vi "CalibrateDistanceCameraSyringe (SubVI).vi"() -> ()   [LabVIEW 2016]
uses:
  <vilib>/LabVIEW Interface for Arduino/Type Defs/Arduino Resource.ctl
  <vilib>/LabVIEW Interface for Arduino/Type Defs/Board Type.ctl
  C:/Users/Aerotech/Documents/BNL_ThermomechanicalStave/AerotechLibraries/Bin/Aerotech.A3200.dll
  AerotechLibraries/Bin/Aerotech.A3200.dll
  <vilib>/vision/Measure.llb/Edge Options.ctl
  <vilib>/vision/Measure.llb/Edge Polarity.ctl
  <vilib>/vision/Image Controls.llb/IMAQ Image.ctl
  <vilib>/LabVIEW Interface for Arduino/Type Defs/Pin Mode.ctl
  <vilib>/LabVIEW Interface for Arduino/LabVIEW Interface for Arduino.lvlib
  <vilib>/vision/NI_Vision_Development_Module.lvlib
panel:
  in  "?":T1(tab)
  in  "Coordinate to Dot":T2={"X [mm]"=10.0, "Y [mm]"=-20.0, "Z [mm] "=43.0}
  in  "Estimate distance x":dbl
  in  "Estimate distance y":dbl
  in  "Camera Z":dbl
  out "XYZ Stage Control":refnum<k24>
  out "Arduino Resource":T3={"VISA resource"="COM3", "Board Type"=enum."Uno", "Connection Type"=enum."USB / Serial", "Bytes Per Packet (15)"=15}
  in  "Digital I/O Pin":u8=7
  in  "Axis speeds (mm/s)":T5={"vX [mm]"=150.0, "vY [mm]"=150.0, "vZ [mm] "=150.0}
  in  "Lowest Z Position":dbl=46.0
  in  "um/pix resolution":dbl=1.5800403213058958
  out "Template Image":T6
  in  "Template Path":path=path "C:/Users/Aerotech/Documents/BNL_ThermomechanicalStave/0_Calibration"
  in  "Circle Finding Options":T9={"Search  Direction"=1, "Edge Options"={"Edge Polarity"=2, "Kernel Size"=3, "Width"=3, "Minimum Edge Strength"=10.0, "Interpolation Type"=enum."Bilinear Fixed", "Data Processing Method"=enum."Median"}, "Show Search Area"=FALSE, "Show Search Lines"=FALSE, "Show Edges Found"=FALSE, "Show Result"=TRUE, "Search Area Color"=65280, "Search Lines Color"=255, "Edge Locations Color"=16776960, "Result Color"=65511, "Overlay Group Name"=""} {"Search  Direction" items=["Outside to Inside", "Inside to Outside"]; "Edge Options"."Edge Polarity" items=["All Edges", "Rising Edges", "Falling Edges"]; "Edge Options"."Minimum Edge Strength" format="%.2f"; "Edge Options"."Width" step=2; "Edge Options"."Kernel Size" step=2}
  in  "Circle ROI Descriptor":T10={"Global Rectangle"=[675, 567, 1751, 1642], "Contours"=[{"ID"=enum."External", "Type"=7, "Coordinates"=[1212, 1104, 85, 537, 0, 0]}]} {"Contours"."Type" items=["No Selection", "Point", "Line", "Rectangle", "Oval", "Polygon", "Freehand Region", "Annulus", "Unused2", "Unused3", "Broken Line", "Freehand Line", "Rotated Rectangle"]}
  in  "Pattern Match Settings":T11={"Algorithm"=2, "Number of Matches Requested"=1, "Minimum Match Score"=700.0, "SubPixel Accuracy"=TRUE, "Rotation Angle Ranges"=[{"Start"=0.0, "End"=360.0}], "Show Search Area"=FALSE, "Show Result"=TRUE} {"Rotation Angle Ranges"."End" format="%.1f"; "Rotation Angle Ranges"."Start" format="%.1f"; "Minimum Match Score" min=0 max=1000 format="%.2f"; "Number of Matches Requested" min=1; "Algorithm" items=["All", "Low Discrepancy Sampling", "Grayscale Value Pyramid", "Gradients Pyramid"]}
  in  "Circle Fit Options":T12={"Process"=enum."Get Best Edge", "Step Size"=3.0, "Max Pixel Radius"=3}
  out "Estimate location":T2={"X [mm]"=10.0, "Y [mm]"=-20.0, "Z [mm] "=43.0}
  out "X/Y difference (CAMERA - SYRINGE)":dbl[](array[numeric])
  out "error out":errorcluster
  out "pixels x":dbl=1920.0
  out "pixels y":dbl=1374.0
  out "Dot image":T6(plugin-control)
  in  "error in":errorcluster
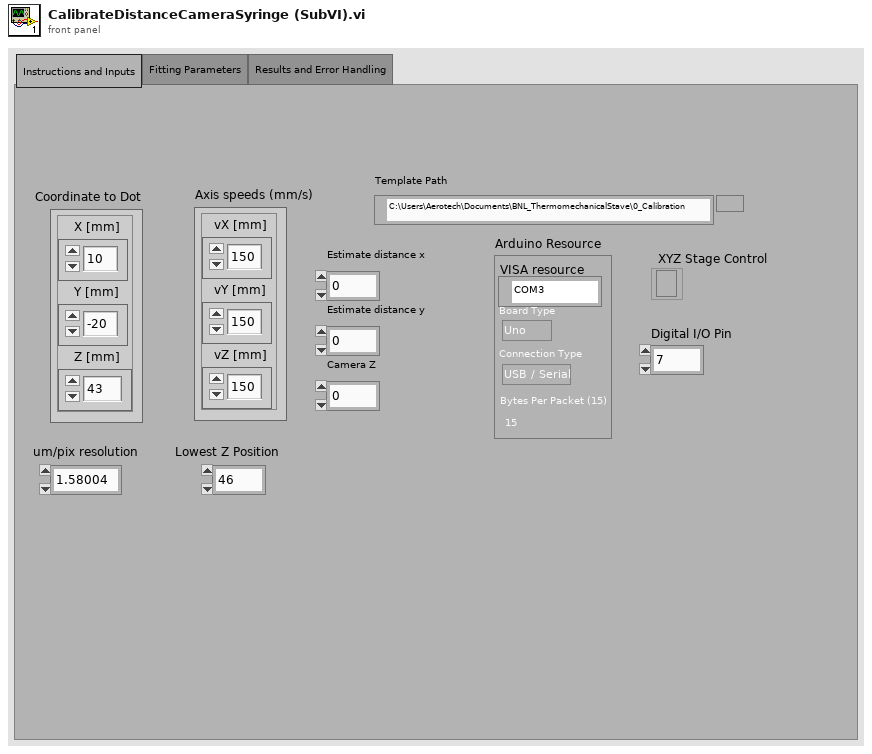
[diagram p1: front panel]
types:
  T1 = enum32{"Instructions and Inputs", "Fitting Parameters", "Results and Error Handling"}
  T2 = cluster{"X [mm]":dbl, "Y [mm]":dbl, "Z [mm] ":dbl}
  T3 = typedef "LabVIEW Interface for Arduino.lvlib/Arduino Resource.ctl" = cluster{"VISA resource":refnum<visa-resource-name>, "Board Type":T4, "Connection Type":enum8{"USB / Serial"}, "Bytes Per Packet (15)":u8}
  T4 = typedef "LabVIEW Interface for Arduino.lvlib/Board Type.ctl" = enum16{"Uno", "Dimuelanove w/Atmega 328", "Mega 2560"}
  T5 = cluster{"vX [mm]":dbl, "vY [mm]":dbl, "vZ [mm] ":dbl}
  T6 = typedef "IMAQ Image.ctl" = refnum<image>
  T7 = typedef "Edge Options.ctl" = cluster{"Edge Polarity":T8, "Kernel Size":u32, "Width":u32, "Minimum Edge Strength":sgl, "Interpolation Type":enum32{"Zero Order", "Bilinear", "Quadratic", "Cubic", "Bilinear Fixed"}, "Data Processing Method":enum32{"Average", "Median"}}
  T8 = typedef "Edge Polarity.ctl" = u32
  T9 = cluster{"Search  Direction":u32, "Edge Options":T7, "Show Search Area":bool, "Show Search Lines":bool, "Show Edges Found":bool, "Show Result":bool, "Search Area Color":u32, "Search Lines Color":u32, "Edge Locations Color":u32, "Result Color":u32, "Overlay Group Name":string}
  T10 = cluster{"Global Rectangle":i32[], "Contours":cluster{"ID":enum32{"External", "Internal"}, "Type":u32, "Coordinates":i32[]}[]}
  T11 = cluster{"Algorithm":i32, "Number of Matches Requested":i32, "Minimum Match Score":sgl, "SubPixel Accuracy":bool, "Rotation Angle Ranges":cluster{"Start":sgl, "End":sgl}[], "Show Search Area":bool, "Show Result":bool}
  T12 = cluster{"Process":enum16{"Get First Edge", "Get First + Last Edge", "Get All Edges", "Get Best Edge"}, "Step Size":dbl, "Max Pixel Radius":i32}
  T13 = typedef "Image Type" = u32
  T14 = typedef "LabVIEW Interface for Arduino.lvlib/Pin Mode.ctl" = enum8{"Input", "Output"}
  T15 = cluster{"Final X":dbl, "Final Y":dbl, "Final Z":dbl}
  T16 = cluster{"X [mm]":dbl, "Y [mm]":dbl, "Lowest Z Position":dbl}
  T17 = cluster{"Position":cluster{"x":sgl, "y":sgl}, "Angle":sgl, "Scale":sgl, "Score":sgl, "Bounding Box":cluster{"x":sgl, "y":sgl}[]}[]
  T18 = cluster{"Global Rectangle":i32[], cluster{"ID":enum32{"External", "Internal"}, "Type":u32, "Coordinates":i32[]}[]}
  T19 = cluster{"Center (Pixels)":cluster{"X":sgl, "Y":sgl}, "Radius (Pixels)":dbl, "Center (Real-World)":cluster{"X":sgl, "Y":sgl}, "Radius (Real-World)":dbl, "Roundness (Real-World)":dbl, "Average Strength":dbl, "Average SNR (dB)":dbl}
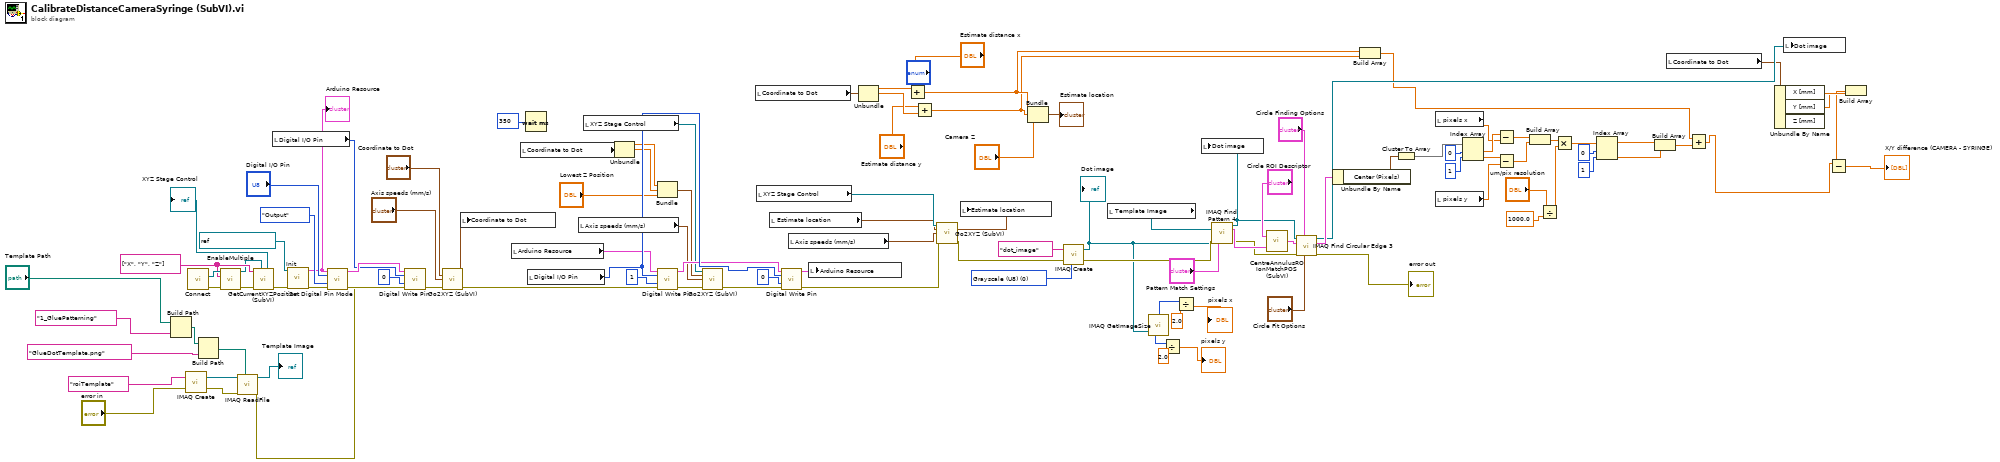
[diagram p0: block diagram]
diagram:
  w64 = T13 0 items=["Grayscale (U8)", "Grayscale (I16)", "Grayscale (SGL)", "Complex (CSG)", "RGB (U32)", "HSL (U32)", "RGB (U64)", "Grayscale (U16)"] ("Image Type")
  w100 = string[] ["X", "Y", "Z"] ("Axes Names")
  n1 = Build Path(base path="Template Path", name or relative path="1_GluePatterning") -> (appended path=w9:path)
  n2 = call "IMAQ Create"("Image Name"="roiTemplate", "error in (no error)"="error in") -> ("New Image"=w12:T6, "error out"=w13:errorcluster)  [unwired: 3 in]
  n3 = Build Path(base path=w9, name or relative path="GlueDotTemplate.png") -> (appended path=w7:path)
  n4 = call "IMAQ ReadFile"("File Path"=w7, "error in (no error)"=w13, "Image"=w12) -> ("error out"=w4:errorcluster, "Image Out"=→"Template Image":T6)  [unwired: 4 in, 3 out]
  n5 = call "Connect.vi"("error in (no error)"=w4) -> ("error out"=w102:errorcluster, "controller"=w101:refnum<k24>)  [unwired: 9 in]
  n6 = call "EnableMultiple.vi"("error in (no error)"=w102, "axis names"=w100, "controller in"=w101) -> ("error out"=w103:errorcluster, "controller out"=w99:refnum<k24>)  [unwired: 7 in]
  n7 = call "GetCurrentXYZPosition (SubVI).vi"(".NET Refnum in - Device"=w99, "error in (no error)"=w103, "Axes Names"=w100) -> ("error out"=w97:errorcluster, ".NET Refnum out  - Device"=→"XYZ Stage Control":refnum<k24>)  [unwired: 3 in, 4 out]
  n8 = local read "Digital I/O Pin"() -> (w105:u8)
  n9 = call <vilib>:"Init.vi"("VISA resource"=refnum<visa-resource-name> "COM3", "error in"=w97) -> ("Arduino Resource"=w104:T3, "error out"=w106:errorcluster)  [unwired: 16 in]
  "Arduino Resource" <- w104
  n10 = call <vilib>:"Set Digital Pin Mode.vi"("Arduino Resource"=w104, "Digital I/O Pin"="Digital I/O Pin", "Pin Mode (Input)"=Pin_Mode."Output", "error in"=w106) -> ("Arduino Resource"=w109:T3, "error out"=w110:errorcluster)  [unwired: 10 in]
  n11 = call <vilib>:"Digital Write Pin.vi"("Arduino Resource"=w109, "Digital I/O Pin (0)"=w105, "Value (0)"=u8 0, "error in"=w110) -> ("error out"=w94:errorcluster)  [unwired: 10 in, 1 out]
  n12 = call "Go2XYZ (SubVI).vi"("Go to Coordinates"="Coordinate to Dot", "Axis Speeds"="Axis speeds (mm/s)", "error in (no error)"=w94) -> ("Final Position"=w61:T15, "error out"=w90:errorcluster)  [unwired: 8 in, 3 out]
  n13 = local write "Coordinate to Dot"(w61) -> ()
  n14 = local read "Arduino Resource"() -> (w82:T3)
  n15 = local read "Coordinate to Dot"() -> (w85:T2)
  n16 = Wait (ms)(milliseconds to wait=u32 350) -> ()  [unwired: 1 out]
  n17 = local read "Digital I/O Pin"() -> (w92:u8)
  n18 = local read "Axis speeds (mm/s)"() -> (w88:T5)
  n19 = local read "XYZ Stage Control"() -> (w87:refnum<k24>)
  n20 = Unbundle(w85) -> ("X [mm]"=w84:dbl, "Y [mm]"=w83:dbl)  [unwired: 1 out]
  n21 = Bundle("X [mm]"=w84, "Y [mm]"=w83, "Lowest Z Position"="Lowest Z Position") -> (w86:T16)  [unwired: 1 in]
  n22 = call <vilib>:"Digital Write Pin.vi"("Arduino Resource"=w82, "Digital I/O Pin (0)"=w92, "Value (0)"=u8 1, "error in"=w90) -> ("Arduino Resource"=w91:T3, "error out"=w80:errorcluster)  [unwired: 10 in]
  n23 = call "Go2XYZ (SubVI).vi"(".NET Refnum in"=w87, "Go to Coordinates"=w86, "Axis Speeds"=w88, "error in (no error)"=w80) -> ("error out"=w93:errorcluster)  [unwired: 7 in, 4 out]
  n24 = local read "Coordinate to Dot"() -> (w78:T2)
  n25 = local read "XYZ Stage Control"() -> (w76:refnum<k24>)
  n26 = local read "Estimate location"() -> (w67:T2)
  n27 = call <vilib>:"Digital Write Pin.vi"("Arduino Resource"=w91, "Digital I/O Pin (0)"=w92, "Value (0)"=u8 0, "error in"=w93) -> ("Arduino Resource"=w74:T3, "error out"=w73:errorcluster)  [unwired: 10 in]
  n28 = local read "Axis speeds (mm/s)"() -> (w77:T5)
  n29 = local write "Arduino Resource"(w74) -> ()
  n30 = Unbundle(w78) -> ("X [mm]"=w72:dbl, "Y [mm]"=w71:dbl)  [unwired: 1 out]
  n31 = Add(x=w72, y="Estimate distance x") -> (x+y=w30:dbl)
  n32 = Add(x="Estimate distance y", y=w71) -> (x+y=w29:dbl)
  n33 = call "Go2XYZ (SubVI).vi"(".NET Refnum in"=w76, "Go to Coordinates"=w67, "Axis Speeds"=w77, "error in (no error)"=w73) -> ("Final Position"=w60:T15, "error out"=w65:errorcluster)  [unwired: 7 in, 3 out]
  n34 = local write "Estimate location"(w60) -> ()
  n35 = Bundle(w30, w29, "Camera Z"="Camera Z") -> (→"Estimate location":cluster{dbl, dbl, "Camera Z":dbl})  [unwired: 1 in]
  n36 = call "IMAQ Create"("Image Name"="dot_image", "Image Type"=w64, "error in (no error)"=w65) -> ("New Image"=w21:T6, "error out"=w62:errorcluster)  [unwired: 1 in, 1 out]
  "Dot image" <- w21
  n37 = local read "Template Image"() -> (w2:T6)
  n38 = call "IMAQ GetImageSize"("Image"=w21) -> ("Y Resolution"=w26:i32, "X Resolution"=w23:i32)  [unwired: 3 in, 1 out]
  n39 = Divide(x=w26, y=2.0) -> (x/y=→"pixels y":dbl)
  n40 = Divide(x=w23, y=2.0) -> (x/y=→"pixels x":dbl)
  n41 = call "IMAQ Find Pattern 4"("Image"=w21, "Template"=w2, "error in"=w62, "Settings"="Pattern Match Settings") -> ("Image Out"=w34:T6, "Matches (pixel)"=w33:T17, "error out"=w32:errorcluster)  [unwired: 5 in, 4 out]
  n42 = local write "Dot image"(w34) -> ()
  n43 = call "CentreAnnulusROIonMatchPOS (SubVI).vi"("Matches (pixel)"=w33, "Annulus ROI Descriptor"="Circle ROI Descriptor") -> ("Annulus ROI Descriptor centred on match position"=w53:T18)
  n44 = call "IMAQ Find Circular Edge 3"("Circle Fit Options"="Circle Fit Options", "Options"="Circle Finding Options", "error in (no error)"=w32, "ROI Descriptor"=w53, "Image"=w34) -> ("error out"=→"error out":errorcluster, "Fitted Circle"=w48:T19, "Image Out"=w31:T6)  [unwired: 2 in, 2 out]
  n45 = Unbundle By Name(w48) -> ("Center (Pixels)"=w38:cluster{"X":sgl, "Y":sgl})
  n46 = Build Array(w30, w29) -> (w28:dbl[])
  n47 = Cluster To Array(cluster=w38) -> (array=w44:sgl[])
  n48 = local read "pixels x"() -> (w39:dbl)
  n49 = local read "pixels y"() -> (w40:dbl)
  n50 = Index Array(array=w44, index #1=0 ("index"), index #2=1 ("index")) -> (element #1=w45:sgl, element #2=w41:sgl)
  n51 = Subtract(x=w45, y=w39) -> (x-y=w47:dbl)
  n52 = Subtract(x=w41, y=w40) -> (x-y=w46:dbl)
  n53 = Build Array(w47, w46) -> (w37:dbl[])
  n54 = Divide(x="um/pix resolution", y=1000.0) -> (x/y=w50:dbl)
  n55 = Multiply(x=w37, y=w50) -> (x*y=w57:dbl[])
  n56 = Index Array(array=w57, index #1=0, index #2=1) -> (element #1=w36:dbl, element #2=w35:dbl)
  n57 = Build Array(w36, w35) -> (w49:dbl[])
  n58 = local read "Coordinate to Dot"() -> (w20:T2)
  n59 = Add(x=w28, y=w49) -> (x+y=w16:dbl[])
  n60 = Unbundle By Name(w20) -> ("X [mm]"=w19:dbl, "Y [mm]"=w18:dbl)  [unwired: 1 out]
  n61 = local write "Dot image"(w31) -> ()
  n62 = Build Array(w19, w18) -> (w17:dbl[])
  n63 = Subtract(x=w16, y=w17) -> (x-y=→"X/Y difference (CAMERA - SYRINGE)":dbl[])
